vi "3.vi"() -> ()   [LabVIEW 2019]
uses:
  <vilib>/imath/engines/lvmath/Plug In/_Char/NIMS_CH_character datatype.ctl
  <vilib>/imath/engines/lvmath2/RunTimeEngine/Managers/WorkSpace/UID Generator.vi
  Documents/LabVIEW Data/MathScriptVIs/MCStatic_41946317732_4cebf1f89a27c07d4b0018885964fd98.vi
  <instcachedir>/0/MCStatic_41946317732_4cebf1f89a27c07d4b0018885964fd98_375143F873F347B0A4F249DD85AD4583.lvgen/MCStatic_41946317732_4cebf1f89a27c07d4b0018885964fd98_375143F873F347B0A4F249DD85AD4583_001.vi
  <vilib>/imath/engines/lvmath2/RunTimeEngine/BuiltInFunctions/crosscorr/NIMS_crosscorr(GM,Str).vi
  <instcachedir>/0/NIMS_crosscorr(GM,Str)_7E3A3CE9917B451394D0C3CD4C3D6955.lvgen/NIMS_crosscorr(GM,Str)_7E3A3CE9917B451394D0C3CD4C3D6955_001.vi
  <vilib>/imath/engines/lvmath2/RunTimeEngine/BuiltInFunctions/crosscorr/NIMS_crosscorr(GV,GV,Str).vi
  <instcachedir>/0/NIMS_crosscorr(GV,GV,Str)_5CA32AC90D1E45F7ACA32A74C95143DE.lvgen/NIMS_crosscorr(GV,GV,Str)_5CA32AC90D1E45F7ACA32A74C95143DE_000.vi
  <vilib>/imath/engines/lvmath2/RunTimeEngine/BuiltInFunctions/figure/NIMS_figure.vi
  <vilib>/imathl/engines/lvmath/Functions/Error Handling/Create Error.vi
  <vilib>/imath/engines/lvmath2/RunTimeEngine/BuiltInFunctions/subplot/NIMS_subplot(I32, I32, I32).vi
  <vilib>/imath/engines/lvmath2/RunTimeEngine/BuiltInFunctions/plot/NIMS_plot(RM, RM, Str).vi
  <vilib>/imath/engines/lvmath/Plug In/_Char/NIMS_CH_Character RV to String.vi
  <vilib>/imath/engines/lvmath2/RunTimeEngine/BuiltInFunctions/title/NIMS_title.vi
  <vilib>/imath/engines/lvmath2/RunTimeEngine/BuiltInFunctions/hold/NIMS_hold(Enums).vi
  <vilib>/imath/engines/lvmath2/RunTimeEngine/Managers/SymbolTable/Clear UID.vi
  <vilib>/imath/engines/lvmath2/RunTimeEngine/NodeEndStatement/NIMS_NodeEndStatement_Output.vi
  <instcachedir>/0/NIMS_NodeEndStatement_Output_53EC0D466D134D7ABD903AC30B43404B.lvgen/NIMS_NodeEndStatement_Output_53EC0D466D134D7ABD903AC30B43404B_000.vi
  <vilib>/imath/engines/lvmath2/RunTimeEngine/ErrorHandling/NIMS_Finalize Error.vi
  Documents/LabVIEW Data/rnd2.m
  <vilib>/imath/engines/lvmath2/RunTimeEngine/Managers/SymbolTable/NIMS_WorkSpace.lvlib
panel:
  out "Rs1s2":dbl[](graph)
  out "Rs2":dbl[][](graph)
  out "Rs1":dbl[][](graph)
  in  "num":dbl
  in  "var2":dbl
  in  "mn2":dbl
  in  "var1":dbl
  in  "mn1":dbl
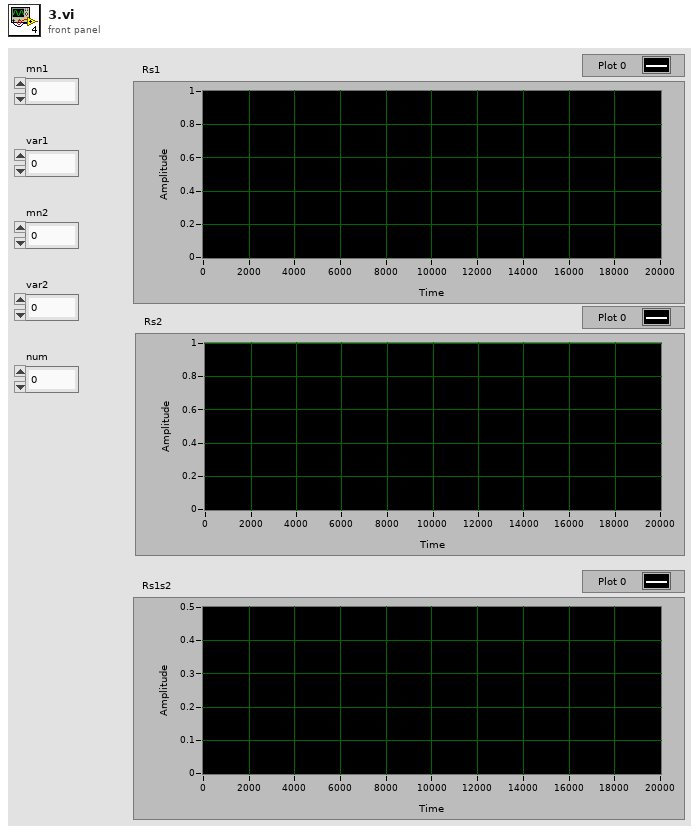
[diagram p1: front panel]
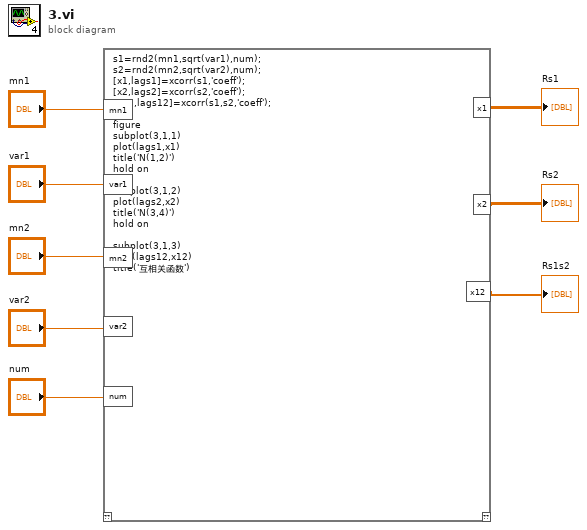
[diagram p0: block diagram]
diagram:
  n1 = mathscript code="s1=rnd2(mn1,sqrt(var1),num);\ns2=rnd2(mn2,sqrt(var2),num);\n[x1,lags1]=xcorr(s1,'coeff');\n[x2,lags2]=xcorr(s2,'coeff');\n[x12,lags12]=xcorr(s1,s2,'coeff');\n\nfigure\nsubplot(3,1,1)\nplot(lags1,x1)\ntitle('N(1,2)')\nhold on\n\nsubplot(3,1,2)\nplot(lags2,x2)\ntitle('N(3,4)')\nhold on\n\nsubplot(3,1,3)\nplot(lags12,x12)\ntitle('互相关函数')"("mn1"="mn1", "var1"="var1", "mn2"="mn2", "var2"="var2", "num"="num") -> ("x1"=→"Rs1":cdb[][], "x2"=→"Rs2":cdb[][], "x12"=→"Rs1s2":cdb[])  [unwired: 1 in, 1 out]
